vi "Lateral Profile.vi"(5 "Lat.Y-Locations":dbl[](array[numeric])=[-500.0, -400.0, -300.0, -200.0, -100.0, 0.0, 100.0, 200.0, 300.0, 400.0, 500.0], 6 "Averaging time (min)":dbl, 7 "Coords":T1, 10 "Tunnel Speed":dbl, 11 "Input Task Array":T4(array[cluster])) -> (3 "Output Task Array":T4(array[cluster]))   [LabVIEW 2015]
uses:
  Anemometry Sub Vis/Gen Trav/Spacing.ctl
  Anemometry Sub Vis/Controls/Multi_run_mode.ctl
  MRCMDFBGlobal.vi
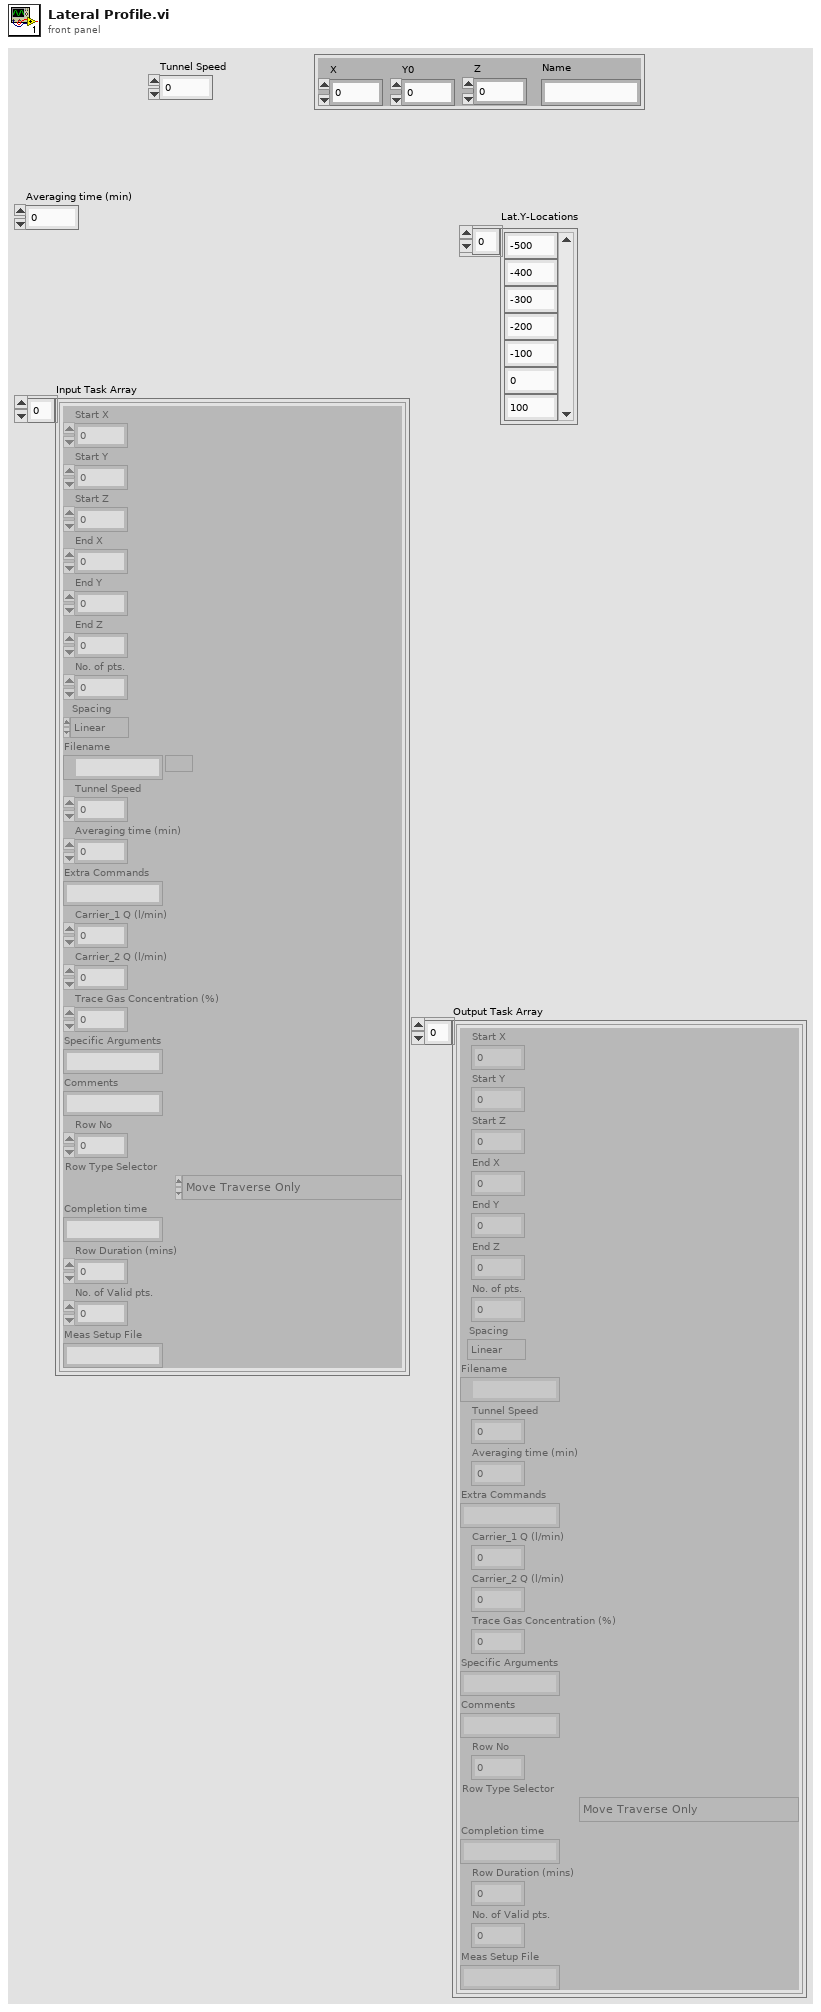
[diagram p1: front panel]
types:
  T1 = cluster{"X":dbl, "Y0":dbl, "Z":dbl, "Name":string}
  T2 = typedef "Spacing.ctl" = enum16{"Linear", "Log", "Gauss", "Specified", "N/A"}
  T3 = typedef "Multi_run_mode.ctl" = enum16{"Move Traverse Only", "Set Tunnel Speed Only", "Set Source Only", "Set Measurement Conditions", "Single Measurement", "Vertical Profile", "Lateral Profile", "Longitudinal Profile", "Explore Volume", "Multi-Axis Profile", "Auto Calibrate", "Meas Fast FID Bkgnd", "Check Beam Power", "Scanning Valve Measurement", "Run VI Named:", "Set ADAM Ch", "Wait (minutes)", "Send Message", "Synchronize With:", "Fall Back to this Row", "Turn Off Row Repeating", "Blank Row", "Traverse 3D Volume"}
  T4 = cluster{"Start X":sgl, "Start Y":sgl, "Start Z":sgl, "End X":sgl, "End Y":sgl, "End Z":sgl, "No. of pts.":i32, "Spacing":T2, "Filename":path, "Tunnel Speed":dbl, "Averaging time (min)":dbl, "Extra Commands":string, "Carrier_1 Q (l/min)":dbl, "Carrier_2 Q (l/min)":dbl, "Trace Gas Concentration (%)":dbl, "Specific Arguments":string, "Comments":string, "Row No":i32, "Row Type Selector":T3, "Completion time":string, "Row Duration (mins)":dbl, "No. of Valid pts.":i32, "Meas Setup File":string}[]
  T5 = cluster{"Start X":sgl, "Start Y":sgl, "Start Z":sgl, "End X":sgl, "End Y":sgl, "End Z":sgl, "No. of pts.":i32, "Spacing":T2, "Filename":path, "Tunnel Speed":dbl, "Averaging time (min)":dbl, "Extra Commands":string, "Carrier_1 Q (l/min)":dbl, "Carrier_2 Q (l/min)":dbl, "Trace Gas Concentration (%)":dbl, "Specific Arguments":string, "Comments":string, "Row No":i32, "Row Type Selector":T3, "Completion time":string, "Row Duration (mins)":dbl, "No. of Valid pts.":i32, "Meas Setup File":string}
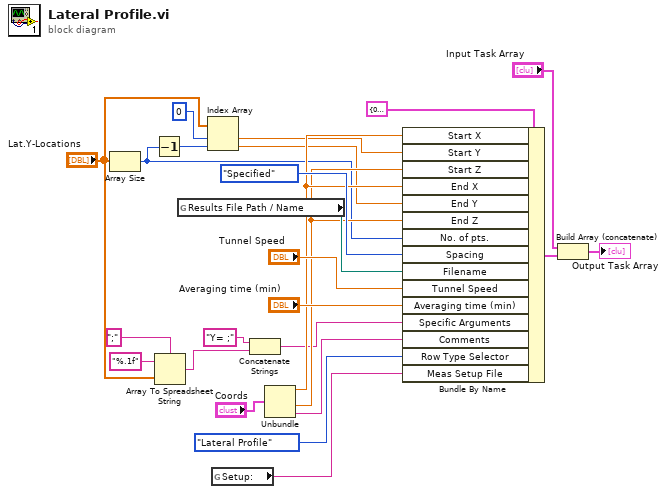
[diagram p0: block diagram]
diagram:
  n1 = Array Size(array="Lat.Y-Locations") -> (size(s)=w1:i32)
  n2 = Decrement(x=w1) -> (x-1=w12:i32)
  n3 = Array To Spreadsheet String(delimiter (Tab)=";", array="Lat.Y-Locations", 3:"%.1f" ("format string")) -> (spreadsheet string=w11:string)
  n4 = global read "MRCMDFBGlobal.vi" "Results File Path / Name"() -> (w16:path)
  n5 = Index Array(array="Lat.Y-Locations", index #1=0 ("index"), index #2=w12) -> (element #1=w3:dbl, element #2=w2:dbl)
  n6 = global read "MRCMDFBGlobal.vi" "Setup:"() -> (w17:string)
  n7 = Concatenate Strings("Y= ;", w11) -> (w4:string)
  n8 = Unbundle("Coords") -> ("X"=w7:dbl, "Z"=w6:dbl, "Name"=w5:string)  [unwired: 1 out]
  n9 = Bundle By Name(cluster=T5 {"Start X"=0.0, "Start Y"=0.0, "Start Z"=0.0, "End X"=0.0, "End Y"=0.0, "End Z"=0.0, "No. of pts."=0, "Spacing"=enum."Linear", "Filename"=path "", "Tunnel Speed"=0.0, "Averaging time (min)"=0.0, "Extra Commands"="", "Carrier_1 Q (l/min)"=0.0, "Carrier_2 Q (l/min)"=0.0, "Trace Gas Concentration (%)"=0.0, "Specific Arguments"="", "Comments"="", "Row No"=0, "Row Type Selector"=enum."Move Traverse Only", "Completion time"="", "Row Duration (mins)"=0.0, "No. of Valid pts."=0, "Meas Setup File"=""} ("RowTemplateConst"), "Start X"=w7, "Start Y"=w3, "Start Z"=w6, "End X"=w7, "End Y"=w2, "End Z"=w6, "No. of pts."=w1, "Spacing"=Spacing."Specified", "Filename"=w16, "Tunnel Speed"="Tunnel Speed", "Averaging time (min)"="Averaging time (min)", "Specific Arguments"=w4, "Comments"=w5, "Row Type Selector"=Multi_run_mode."Lateral Profile", "Meas Setup File"=w17) -> (w19:T5)
  n10 = Build Array (concatenate)("Input Task Array", w19) -> (→"Output Task Array":T4)
